vi "Unlock Topic.vi"(8 "error in (no error)":errorcluster, 10 "Publisher ID":string, 11 "Topic in":refnum<class "Topic.lvclass">) -> (0 "error out":errorcluster, 3 "Topic out":refnum<class "Topic.lvclass">)   [LabVIEW 2017, in "Mediator.lvlib" / "Topic.lvclass"]
doc: "<License>\nCopyright © 2017 Composed Systems, LLC | All rights reserved\nwww.composed.io\n\nAuthor: Ethan Stern <ethan.stern@composed.io>\n\nThis software is provided \"AS IS\" WITHOUT WARRANTIES, either express or implied, AND IS FOR EDUCATIONAL PURPOSES ONLY.\n</License>"
uses:
  Topic.lvclass
  Topic.lvclass/Topic.ctl
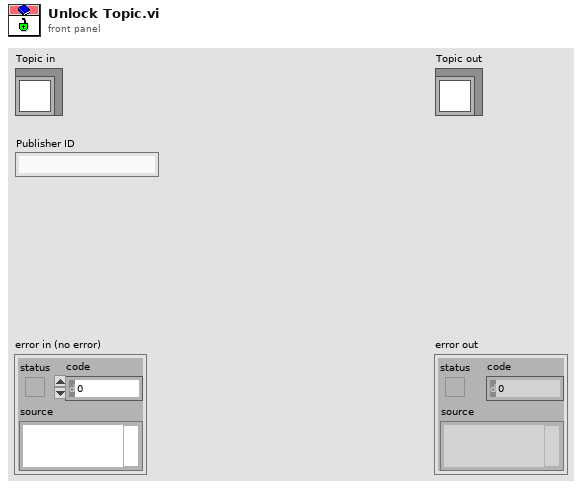
[diagram p1: front panel]
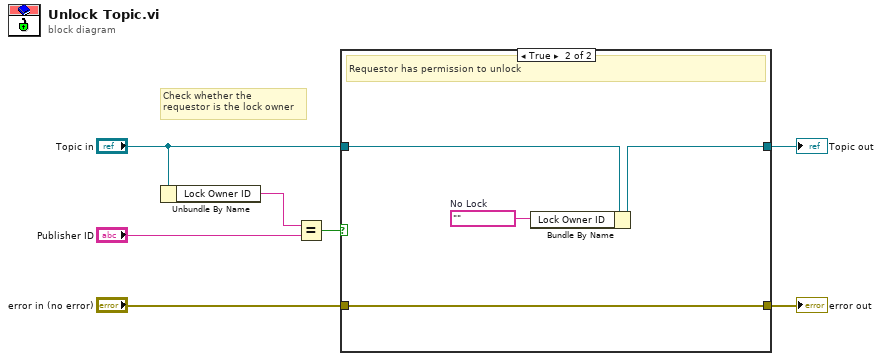
[diagram p0: block diagram]
diagram:
  # "Check whether the\nrequestor is the lock owner"
  n1 = Unbundle By Name("Topic in") -> ("Lock Owner ID"=w2:string)
  n2 = Equal?(x=w2, y="Publisher ID") -> (x = y?=w1:bool)
  n3 = case shown="True" w1 {
    tunnel: "error in (no error)" -> [w9 w11]
    tunnel: [w9 w11] -> w6
    tunnel: [w8 w12] -> w5
    tunnel: "Topic in" -> [w8 w13]
    frame False {
      # "Reject request -- Only the lock holder can unlock"
    }
    frame True {
      w10 = ""  # No Lock
      # "Requestor has permission to unlock"
      n4 = Bundle By Name(cluster=w13, "Lock Owner ID"=w10) -> (w12:refnum<class "Topic.lvclass">)
    }
  }
  "error out" <- w6
  "Topic out" <- w5
